vi "FTW-Scheduler-AddNext.vi"(1 "Add Next in Sequence":string, 3 "FTW Job Scheduler":refnum<class "FTW-Scheduler.lvclass">) -> (0 "FTW Job Scheduler out":refnum<class "FTW-Scheduler.lvclass">)   [LabVIEW 2014, in "FTW-Scheduler.lvclass"]
uses:
  FTW-Scheduler.lvclass
  FTW-Scheduler.lvclass/FTW-Scheduler.ctl
panel:
  # "Inputs"
  # "Outputs"
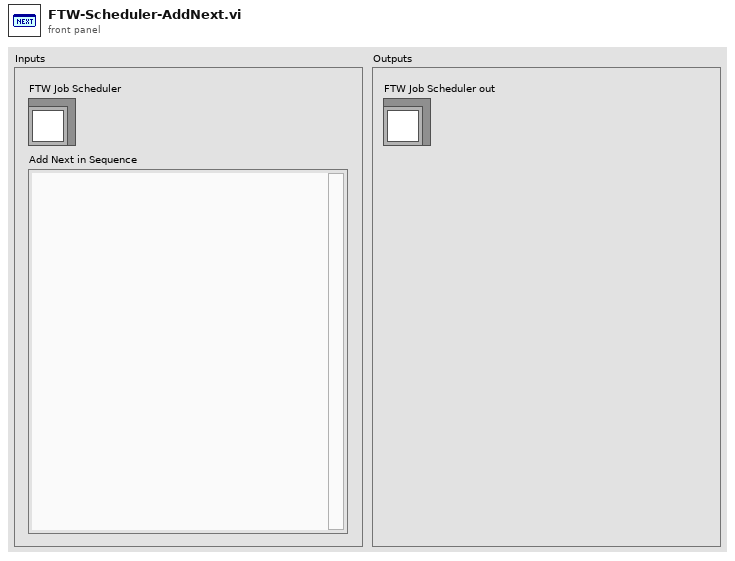
[diagram p1: front panel]
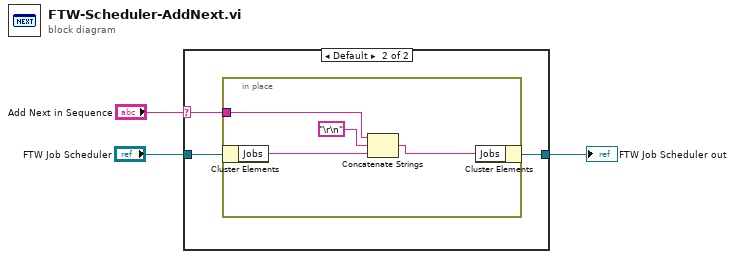
[diagram p0: block diagram]
diagram:
  n1 = case shown="Default" "Add Next in Sequence" {
    selector: "Add Next in Sequence" -> [_ w5]
    tunnel: "FTW Job Scheduler" -> [w4 w7]
    tunnel: [w4 w6] -> w2
    frame "" {
    }
    frame Default {
      n2 = in-place {
        in-place-border: w5 -> [w8]
        n3 = in-place-cluster #1(w7) -> ("Jobs"=w11:string)
        n4 = Concatenate Strings(w8, "\r\n", w11) -> (w9:string)
        n5 = in-place-cluster #1("Jobs"=w9) -> (w6:refnum<class "FTW-Scheduler.lvclass">)
      }
    }
  }
  "FTW Job Scheduler out" <- w2
